vi "Reset Pending Changes.vi"(11 "Data Cluster in":T1) -> (3 "Data Cluster out":T1)   [LabVIEW 2020, in "FrameEditor.lvlib"]
uses:
  FrameEditor.lvlib
  controls/UI Data.ctl
  controls/Type of Payload.ctl
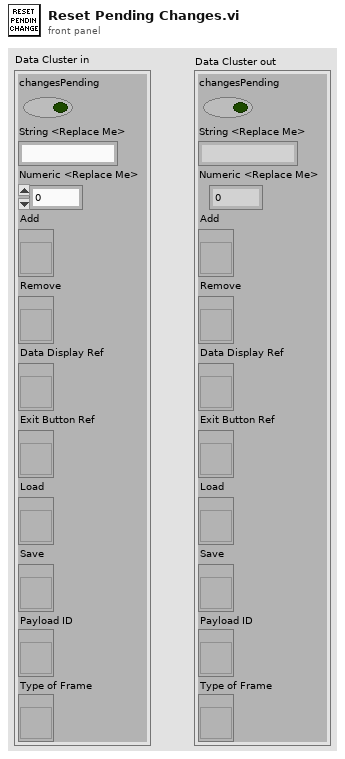
[diagram p1: front panel]
types:
  T1 = typedef "UI Data.ctl" = cluster{"changesPending":bool, "String <Replace Me>":string, "Numeric <Replace Me>":dbl, "Add":refnum<vi>, "Remove":refnum<vi>, "Data Display Ref":refnum<vi>, "Exit Button Ref":refnum<vi>, "Load":refnum<vi>, "Save":refnum<vi>, "Payload ID":refnum<vi>, "Type of Frame":refnum<vi>}
  T2 = enum8{"Enabled", "Disabled", "Disabled and Grayed Out"}
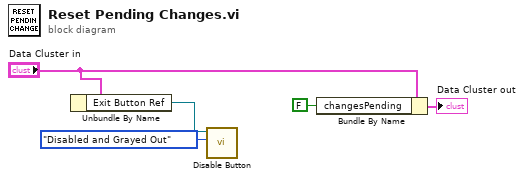
[diagram p0: block diagram]
diagram:
  n1 = Unbundle By Name("Data Cluster in") -> ("Exit Button Ref"=w2:refnum<vi>)
  n2 = call "Disable Button.vi"("Disabled"=T2."Disabled and Grayed Out", "ctrl ref in"=w2) -> ()  [unwired: 10 in]
  n3 = Bundle By Name(cluster="Data Cluster in", "changesPending"=FALSE) -> (→"Data Cluster out":T1)
